vi "test_struct_abs_activity_vapor.vi"() -> ()   [LabVIEW 2017]
doc: "Minimal example that demonstrates functions implemented in the SorpPropLib for absorption working pairs based on the activity approach and using the vapor pressure as additional property."
panel:
  in  "Molar volume of second component in m3/mol (Input)":dbl=-1.0
  in  "Molar volume of first component in m3/mol (Input)":dbl=-1.0
  out "Pressure":cluster{dbl[], dbl[]}[](graph)=[{[1000.0, 1001.0, 1002.0, 1003.0, 1004.0, 1005.0, 1006.0, 1007.0, 1008.0, 1009.0], [-1.0, -1.0, -1.0, -1.0, -1.0, -1.0, -1.0, -1.0, -1.0, -1.0]}, {[1000.0, 1001.0, 1002.0, 1003.0, 1004.0, 1005.0, 1006.0, 1007.0, 1008.0, 1009.0], [-1.0, -1.0, -1.0, -1.0, -1.0, -1.0, -1.0, -1.0, -1.0, -1.0]}]
  out "Mole fraction in liquid phase":cluster{dbl[], dbl[]}[](graph)=[{[1000.0, 1001.0, 1002.0, 1003.0, 1004.0, 1005.0, 1006.0, 1007.0, 1008.0, 1009.0], [-1.0, -1.0, -1.0, -1.0, -1.0, -1.0, -1.0, -1.0, -1.0, -1.0]}, {[1000.0, 1001.0, 1002.0, 1003.0, 1004.0, 1005.0, 1006.0, 1007.0, 1008.0, 1009.0], [-1.0, -1.0, -1.0, -1.0, -1.0, -1.0, -1.0, -1.0, -1.0, -1.0]}]
  in  "WorkingPair (Input)":T1={"no_iso"=1, "no_p_sat"=1, "path_db"="D:\\Driesel\\SorpLibLocal\\labview_wrapper\\data\\json\\sorpproplib.json", "wp_as"="lubricant", "wp_st"="POE", "wp_iso"="WilsonFixedDl", "wp_rf"="R-134a", "rf_rhol"="SaturatedLiquidDensity_EoS1", "no_rhol"=1, "rf_psat"="VaporPressure_EoS1"}
  in  "Temperature in K (Input)":dbl=300.0
  in  "Pressure in Pa (Input)":dbl=1000.0
  # "Increase pressure by 5000 Pa in steps of 1 Pa."
  # "Selecting -1: Constant molar volumes stored in data base are used for calculations!"
  # "Path to database"
  # "Name of sorbent"
  # "Name of sub-type of sorbent"
  # "Name of refrigerant"
  # "Name of isotherm"
  # "ID of isotherm"
  # "Name of calculation approach for vapor pressure"
  # "ID of vapor pressure equation"
  # "Name of calculation approach for liquid density"
  # "ID of liquid density equation"
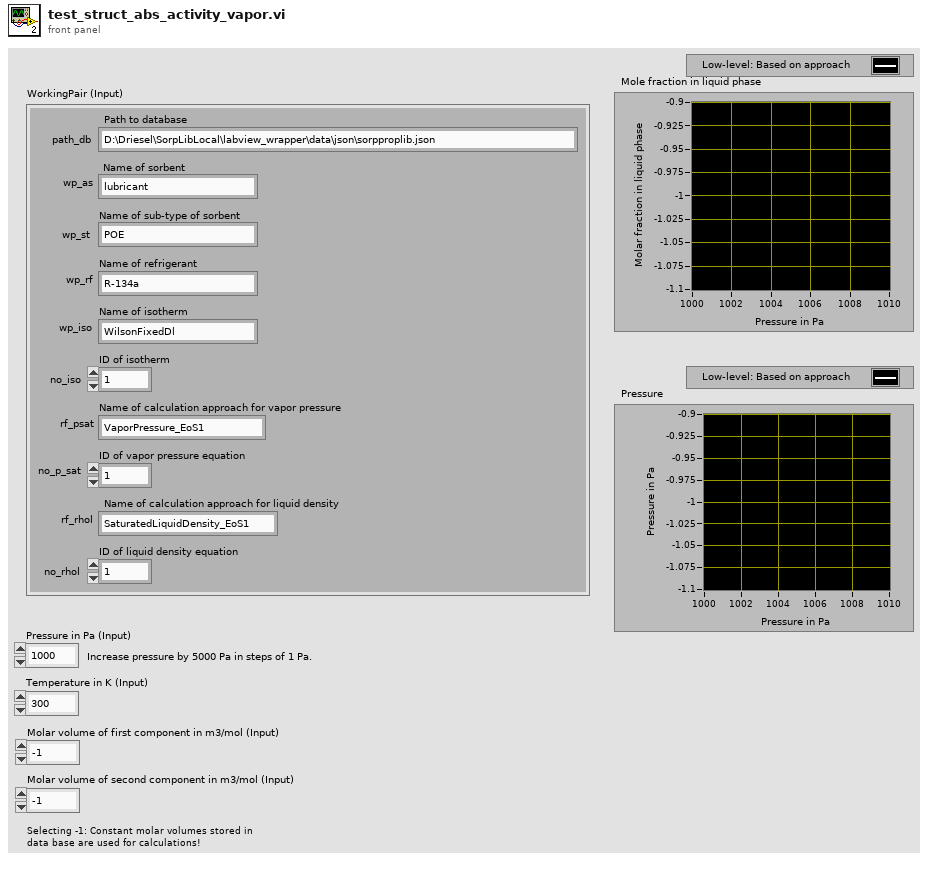
[diagram p1: front panel]
types:
  T1 = cluster{"no_iso":i32, "no_p_sat":i32, "path_db":string, "wp_as":string, "wp_st":string, "wp_iso":string, "wp_rf":string, "rf_rhol":string, "no_rhol":i32, "rf_psat":string}
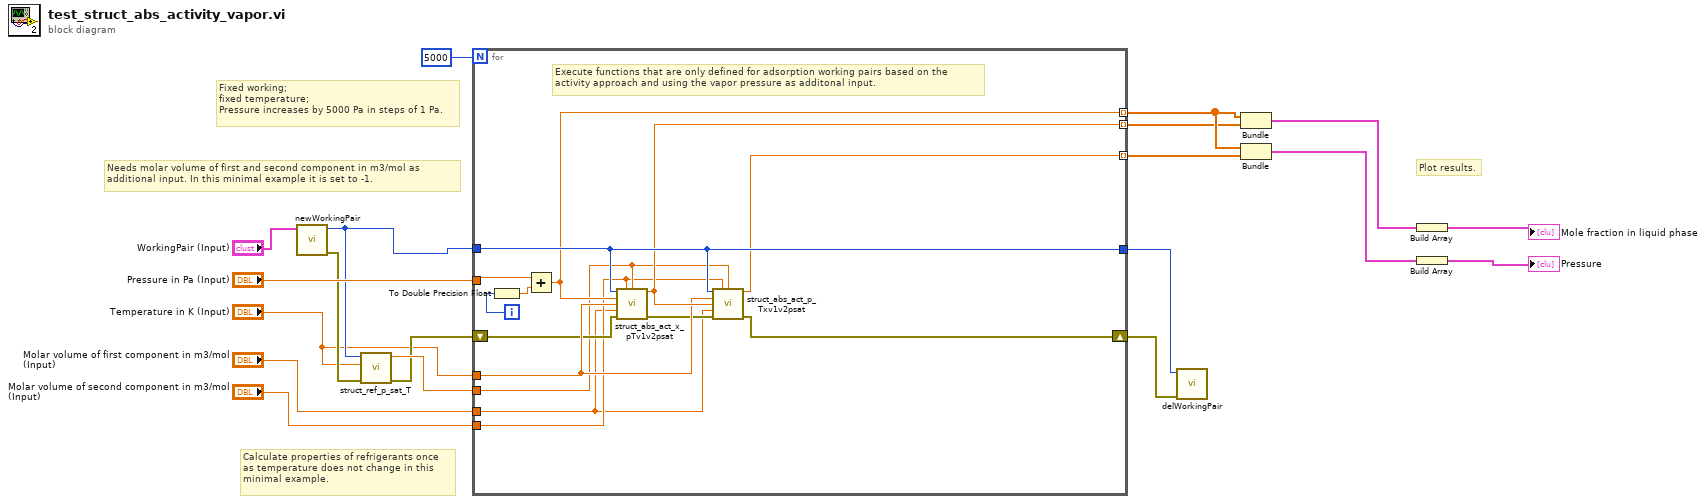
[diagram p0: block diagram]
diagram:
  # "Calculate properties of refrigerants once\nas temperature does not change in this\nminimal example."
  # "Needs molar volume of first and second component in m3/mol as \nadditional input. In this minimal example it is set to -1."
  # "Plot results."
  # "Fixed working;\nfixed temperature;\nPressure increases by 5000 Pa in steps of 1 Pa."
  n1 = call "newWorkingPair.vi"("WorkingPair (Input)"="WorkingPair (Input)") -> ("Error (Output)"=w11:errorcluster, "workingPair"=w10:i64)  [unwired: 9 in]
  n2 = call "struct_ref_p_sat_T.vi"("Error (Input)"=w11, "Temperature in K (Input)"="Temperature in K (Input)", "Reference working pair (Input)"=w10) -> ("Error (Output)"=w7:errorcluster, "Saturation pressure in Pa (Output)"=w12:dbl)  [unwired: 7 in]
  n3 = for {
    N: 5000 -> [_]
    tunnel: "Pressure in Pa (Input)" -> [w33]
    tunnel: "Temperature in K (Input)" -> [w27]
    tunnel: w10 -> [w30]
    shift-right: [w24] -> w13
    shift-left: w7 -> [w26]
    tunnel: [w29] -> w17 mode=indexing
    tunnel: w12 -> [w23]
    tunnel: [w30] -> w9
    tunnel: [w28] -> w8 mode=indexing
    tunnel: [w22] -> w6 mode=indexing
    tunnel: "Molar volume of first component in m3/mol (Input)" -> [w20]
    tunnel: "Molar volume of second component in m3/mol (Input)" -> [w21]
    i -> [w32]
    # "Execute functions that are only defined for adsorption working pairs based on the\nactivity approach and using the vapor pressure as additonal input."
    n4 = To Double Precision Float(number=w32) -> (double precision float=w31:dbl)
    n5 = Add(x=w33, y=w31) -> (x+y=w29:dbl)
    n6 = call "struct_abs_act_x_pTv1v2psat.vi"("Reference working pair (Input)"=w30, "Molar volume of second component in m3/mol (Input)"=w21, "Saturation pressure of first component in Pa (Input)"=w23, "Pressure in Pa (Input)"=w29, "Temperature in K (Input)"=w27, "Molar volume of first component in m3/mol (Input)"=w20, "Error (Input)"=w26) -> ("Mole fraction in liquid phase in mol/mol(Output)"=w28:dbl, "Error (Output)"=w25:errorcluster)  [unwired: 7 in]
    n7 = call "struct_abs_act_p_Txv1v2psat.vi"("Reference working pair (Input)"=w30, "Molar volume of second component in m3/mol (Input)"=w21, "Saturation pressure of first component in Pa (Input)"=w23, "Temperature in K (Input)"=w27, "Mole fraction in liquid phase in mol/mol (Input)"=w28, "Molar volume of first component in m3/mol (Input)"=w20, "Error (Input)"=w25) -> ("Pressure in Pa (Output)"=w22:dbl, "Error (Output)"=w24:errorcluster)  [unwired: 7 in]
  }
  n8 = call "delWorkingPair.vi"("Error (Input)"=w13, "workingPair"=w9) -> ()  [unwired: 9 in, 1 out]
  n9 = Bundle(w17, w8) -> (w16:cluster{dbl[], dbl[]})  [unwired: 1 in]
  n10 = Bundle(w17, w6) -> (w15:cluster{dbl[], dbl[]})  [unwired: 1 in]
  n11 = Build Array(w16) -> (→"Mole fraction in liquid phase":cluster{dbl[], dbl[]}[])
  n12 = Build Array(w15) -> (→"Pressure":cluster{dbl[], dbl[]}[])
